vi "CalcP_Z.vi"(11 "Z[i]":dbl[](graph)) -> (3 "P[i]":dbl[](graph))   [LabVIEW 2018]
uses:
  <vilib>/gmath/NI_Gmath.lvlib
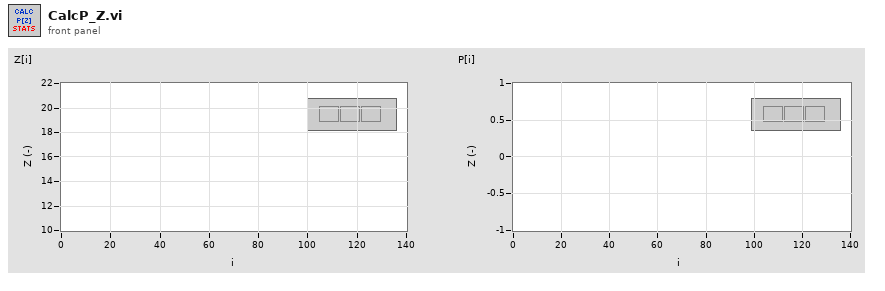
[diagram p1: front panel]
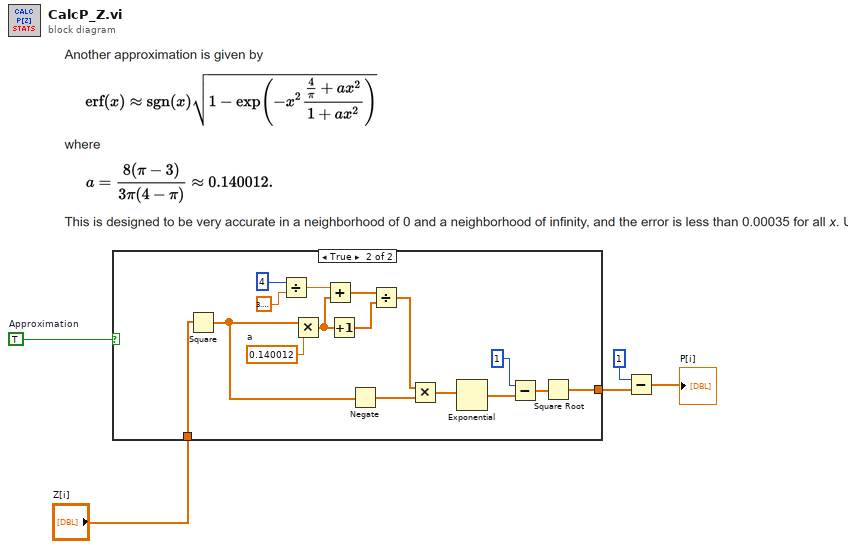
[diagram p0: block diagram]
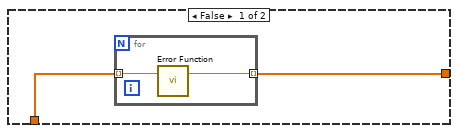
[diagram p2: hidden frame]
diagram:
  w1 = TRUE  # Approximation
  n1 = case shown="True" w1 {
    tunnel: [w6 w12] -> w5
    tunnel: "Z[i]" -> [w7 w10]
    frame False {
      n2 = for {
        tunnel: w7 -> [w9] mode=indexing
        tunnel: [w8] -> w6 mode=indexing
        n3 = call <vilib>:"Error Function.vi"("x"=w9) -> ("erf(x)"=w8:dbl)  [unwired: 2 in]
      }
    }
    frame True {
      w25 = 0.140012  # a
      n4 = Square(x=w10) -> (x^2=w13:dbl[])
      n5 = Divide(x=4, y=3.141592653589793) -> (x/y=w22:dbl)
      n6 = Multiply(x=w13, y=w25) -> (x*y=w21:dbl[])
      n7 = Add(x=w22, y=w21) -> (x+y=w19:dbl[])
      n8 = Increment(x=w21) -> (x+1=w20:dbl[])
      n9 = Negate(x=w13) -> (-x=w17:dbl[])
      n10 = Divide(x=w19, y=w20) -> (x/y=w18:dbl[])
      n11 = Multiply(x=w18, y=w17) -> (x*y=w16:dbl[])
      n12 = Exponential(1:w16) -> (0:w15:dbl[])
      n13 = Subtract(x=1, y=w15) -> (x-y=w14:dbl[])
      n14 = Square Root(x=w14) -> (sqrt(x)=w12:dbl[])
    }
  }
  n15 = Subtract(x=1, y=w5) -> (x-y=→"P[i]":dbl[])
